vi "Do Core.vi"(8 "error in":errorcluster, 9 "Actor in":refnum<class "Actor.lvclass">, 11 "DS Reply Msg in":refnum<class "Reply Msg DataSocket Simple.lvclass">) -> (0 "error out":errorcluster, 1 "Actor out":refnum<class "Actor.lvclass">, 2 "Reply":variant)   [LabVIEW 2023, in "Reply Msg DataSocket Simple.lvclass"]
uses:
  Reply Msg DataSocket Simple.lvclass
  Reply Msg DataSocket Simple.lvclass/Reply Msg DataSocket Simple.ctl
  <vilib>/ActorFramework/Actor/Actor.lvclass
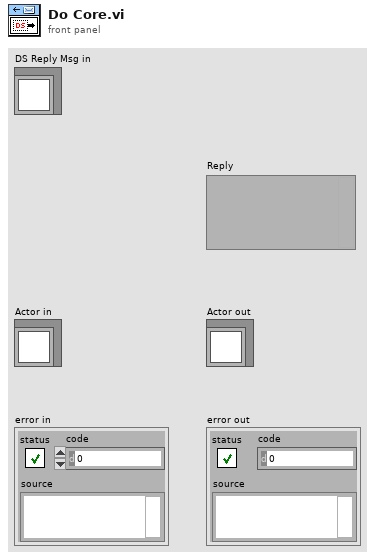
[diagram p1: front panel]
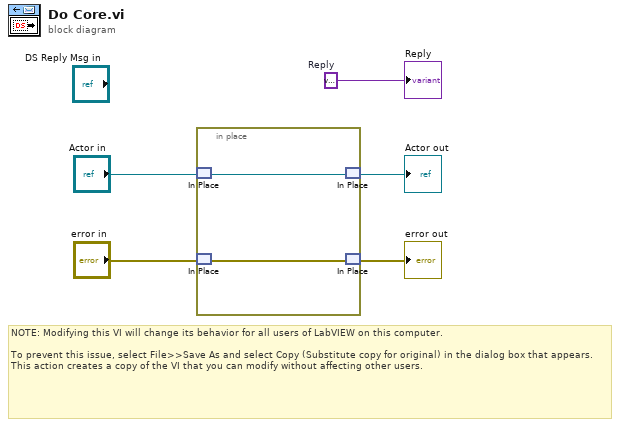
[diagram p0: block diagram]
diagram:
  w1 = variant  # Reply
  # "NOTE: Modifying this VI will change its behavior for all users of LabVIEW on this computer.\n\nTo prevent this issue, select File>>Save As and select Copy (Substitute copy for original) in the dialog box that appears. This action creates a copy of the VI that you can modify without affecting other users."
  n1 = in-place {
    n2 = in-place-match #1("Actor in") -> (w6:refnum<class "Actor.lvclass">)
    n3 = in-place-match #2("error in") -> (w7:errorcluster)
    n4 = in-place-match #1(w6) -> (→"Actor out":refnum<class "Actor.lvclass">)
    n5 = in-place-match #2(w7) -> (→"error out":errorcluster)
  }
  "Reply" <- w1
